vi "Request Data JSON.vi"(8 "error in (no error)":errorcluster, 11 "GetSourceScreenshot in":refnum<class "GetSourceScreenshot.lvclass">) -> (0 "error out":errorcluster, 2 "Request Data JSON":string, 3 "GetSourceScreenshot out":refnum<class "GetSourceScreenshot.lvclass">)   [LabVIEW 2020, in "obs-websocket.lvlib" / "GetSourceScreenshot.lvclass"]
uses:
  GetSourceScreenshot.lvclass
  GetSourceScreenshot.lvclass/GetSourceScreenshot.ctl
  <vilib>/IlluminatedG/lv-web-crypto/lv-json/JSON/JSON.lvlib
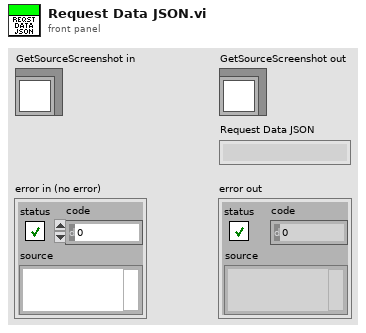
[diagram p1: front panel]
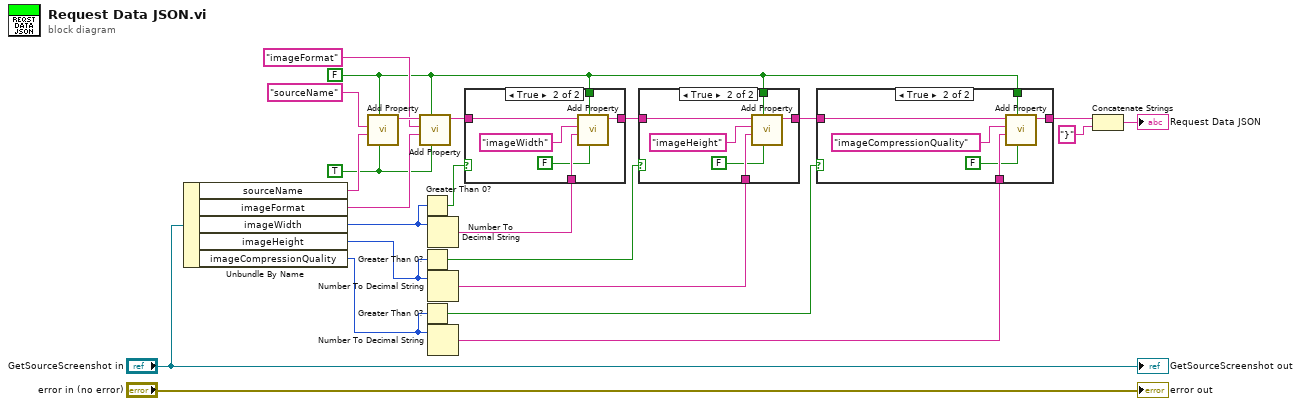
[diagram p0: block diagram]
diagram:
  w17 = TRUE ("String?")
  w4 = FALSE ("Include Empty?")
  n1 = Unbundle By Name("GetSourceScreenshot in") -> ("sourceName"=w21:string, "imageFormat"=w18:string, "imageWidth"=w16:i32, "imageHeight"=w12:i32, "imageCompressionQuality"=w11:i32)
  n2 = call <vilib>:"Add Property.vi"("String?"=w17, "Include Empty?"=w4, "Value"=w21, "Property Name"="sourceName") -> ("String out"=w20:string)  [unwired: 7 in]
  n3 = call <vilib>:"Add Property.vi"("String?"=w17, "Include Empty?"=w4, "Value"=w18, "Property Name"="imageFormat", "String In"=w20) -> ("String out"=w13:string)  [unwired: 6 in]
  n4 = Greater Than 0?(x=w16) -> (x > 0?=w15:bool)
  n5 = Greater Than 0?(x=w12) -> (x > 0?=w9:bool)
  n6 = Greater Than 0?(x=w11) -> (x > 0?=w6:bool)
  n7 = Number To Decimal String(number=w16) -> (decimal integer string=w14:string)  [unwired: 1 in]
  n8 = Number To Decimal String(number=w12) -> (decimal integer string=w8:string)  [unwired: 1 in]
  n9 = Number To Decimal String(number=w11) -> (decimal integer string=w5:string)  [unwired: 1 in]
  n10 = case shown="True" w15 {
    tunnel: w14 -> [_ w31]
    tunnel: w4 -> [_ w29]
    tunnel: w13 -> [w25 w27]
    tunnel: [w25 w26] -> w10
    frame False {
    }
    frame True {
      n11 = call <vilib>:"Add Property.vi"("String?"=FALSE, "Include Empty?"=w29, "Value"=w31, "Property Name"="imageWidth", "String In"=w27) -> ("String out"=w26:string)  [unwired: 6 in]
    }
  }
  n12 = case shown="True" w9 {
    tunnel: w8 -> [_ w38]
    tunnel: w4 -> [_ w36]
    tunnel: w10 -> [w32 w34]
    tunnel: [w32 w33] -> w7
    frame False {
    }
    frame True {
      n13 = call <vilib>:"Add Property.vi"("String?"=FALSE, "Include Empty?"=w36, "Value"=w38, "Property Name"="imageHeight", "String In"=w34) -> ("String out"=w33:string)  [unwired: 6 in]
    }
  }
  n14 = case shown="True" w6 {
    tunnel: w5 -> [_ w45]
    tunnel: w7 -> [w39 w42]
    tunnel: [w39 w41] -> w3
    tunnel: w4 -> [_ w40]
    frame False {
    }
    frame True {
      n15 = call <vilib>:"Add Property.vi"("String?"=FALSE, "Include Empty?"=w40, "Value"=w45, "Property Name"="imageCompressionQuality", "String In"=w42) -> ("String out"=w41:string)  [unwired: 6 in]
    }
  }
  n16 = Concatenate Strings(w3, "}" ("string")) -> (→"Request Data JSON":string)
  "error out" <- "error in (no error)"
  "GetSourceScreenshot out" <- "GetSourceScreenshot in"
